vi "Collide.vi"(9 "Team In":refnum<class "Team.lvclass">, 11 "MySquare in":refnum<class "MySquare.lvclass">) -> (1 "Team":refnum<class "Team.lvclass">, 3 "MySquare out":refnum<class "MySquare.lvclass">)   [LabVIEW 2020, in "SquareTeam.lvlib" / "MySquare.lvclass"]
uses:
  MySquare.lvclass
  SquareBattle/Team/Team.lvclass
  MyTeam/MyTeam.lvclass
  C:/dev/illuminatedg/sol-squarebattle/ProjectTemplates/Source/SummerOfLabVIEW/SquareBattle/template/SquareBattle/Team/Team.lvclass
  MySquare.lvclass/MySquare.ctl
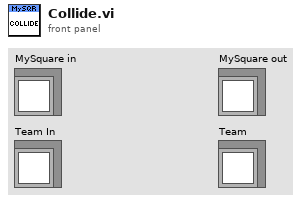
[diagram p1: front panel]
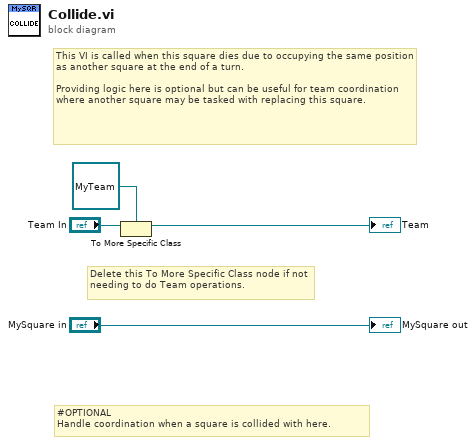
[diagram p0: block diagram]
diagram:
  # "#OPTIONAL\nHandle coordination when a square is collided with here."
  # "Delete this To More Specific Class node if not needing to do Team operations."
  # "This VI is called when this square dies due to occupying the same position as another square at the end of a turn.\n\nProviding logic here is optional but can be useful for team coordination where another square may be tasked with replacing this square."
  n1 = To More Specific Class(target class=refnum<class "MyTeam.lvclass"> refnum ("SquareTeam.lvlib:MyTeam.lvclass"), reference="Team In") -> (specific class reference=→"Team":refnum<class "MyTeam.lvclass">)  [unwired: 1 in, 1 out]
  "MySquare out" <- "MySquare in"
